vi "Just capture.vi"(0 "Camera reference in":refnum<k24>, 5 "Exposure (ms)":dbl=100.0, 11 "Error In":errorcluster) -> (4 "Camera reference out":refnum<k24>, 15 "Error Out":errorcluster)   [LabVIEW 2017]
uses:
  C:/Program Files/National Instruments/LabVIEW 2017/instr.lib/IDS/ueye.NET/uEyeDotNet.dll
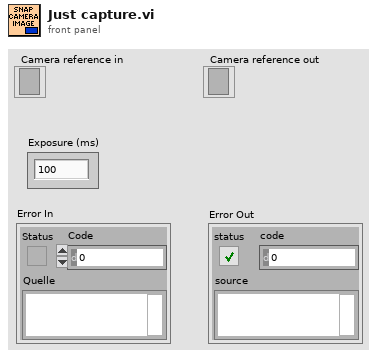
[diagram p1: front panel]
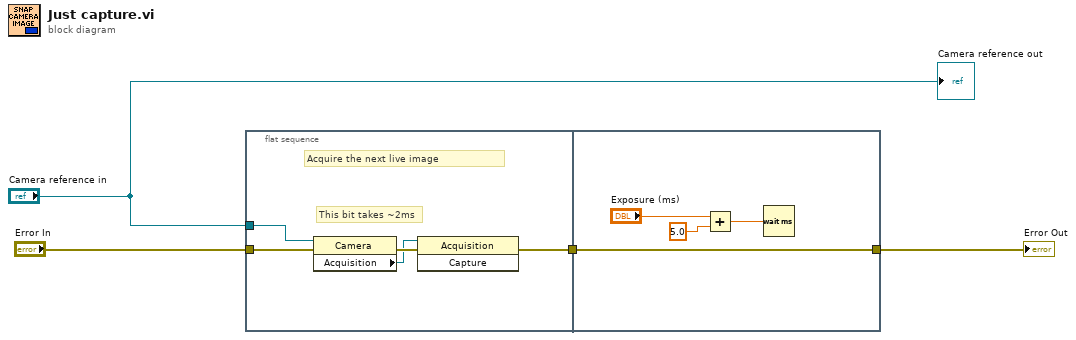
[diagram p0: block diagram]
diagram:
  n1 = flat-sequence {
    tunnel: [w5] -> w1
    tunnel: "Error In" -> [w8]
    tunnel: "Camera reference in" -> [w9]
    tunnel: [w13] -> w4
    tunnel: w1 -> [w13]
    frame #0 {
      # "Acquire the next live image"
      # "This bit takes ~2ms"
      n2 = property class="Camera"(reference=w9, error in=w8) -> (error out=w7:errorcluster, "Acquisition"=w6:refnum<k24>)  [unwired: 1 out]
      n3 = invoke class="Acquisition" method="Capture"(reference=w6, error in=w7) -> (error out=w5:errorcluster)  [unwired: 1 in, 2 out]
    }
    frame #1 {
      n4 = Add(x="Exposure (ms)", y=5.0) -> (x+y=w11:dbl)
      n5 = Wait (ms)(milliseconds to wait=w11) -> ()  [unwired: 1 out]
    }
  }
  "Error Out" <- w4
  "Camera reference out" <- "Camera reference in"
